vi "Config.vi"(8 "error in (no error)":errorcluster, 9 "VISA resource name":refnum<visa-resource-name>, 10 "baud rate":u32=9600, 11 "Serial in":refnum<class "Serial.lvclass">) -> (0 "error out":errorcluster, 3 "Serial out":refnum<class "Serial.lvclass">)   [LabVIEW 2019, in "Serial.lvlib" / "Serial.lvclass"]
uses:
  Serial.lvclass
  Serial.lvclass/Serial.ctl
  <vilib>/Instr/_visa.llb/VISA Configure Serial Port (Instr).vi
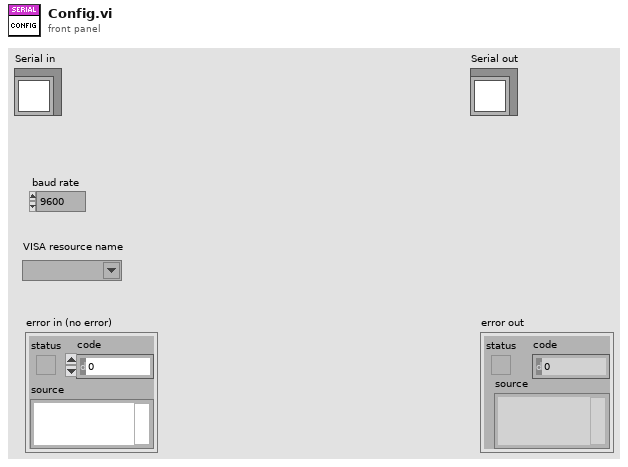
[diagram p1: front panel]
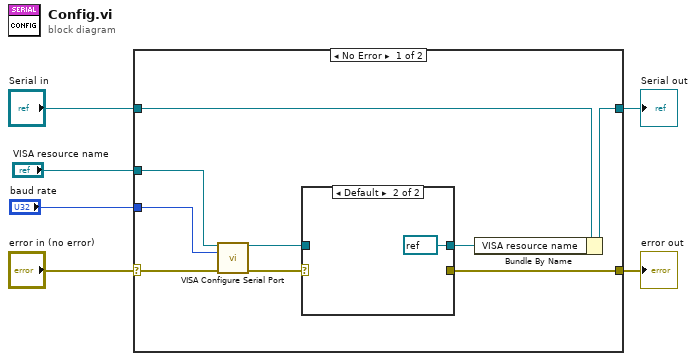
[diagram p0: block diagram]
diagram:
  n1 = case shown="No Error" "error in (no error)" {
    selector: "error in (no error)" -> [w15 w20]
    tunnel: [w11 w20] -> w5
    tunnel: [w10 w19] -> w3
    tunnel: "Serial in" -> [w13 w19]
    tunnel: "VISA resource name" -> [w14 _]
    tunnel: "baud rate" -> [w12 _]
    frame No Error {
      n2 = call-poly "VISA Configure Serial Port"("VISA resource name"=w14, "baud rate (9600)"=w12, "error in (no error)"=w15) -> ("VISA resource name out"=w9:refnum<visa-resource-name>, "error out"=w7:errorcluster)  [unwired: 7 in, 4 out]
      n3 = case shown="Default" w7 {
        selector: w7 -> [w17 _]
        tunnel: [w17 _] -> w11
        tunnel: w9 -> [w16 _]
        tunnel: [w16 refnum<visa-resource-name> refnum ("VISA resource name out")] -> w8
        frame No Error {
        }
        frame Default {
        }
      }
      n4 = Bundle By Name(cluster=w13, "VISA resource name"=w8) -> (w10:refnum<class "Serial.lvclass">)
    }
    frame Error {
    }
  }
  "error out" <- w5
  "Serial out" <- w3
